vi "Main_C8855-01.vi"() -> ()   [LabVIEW 2017]
uses:
  C8855_MainD.ctl
  C8855-01api.dll
panel:
  in  "TrgEdge":u8(ring) caption="Trigger Edge"
  in  "TrgMode":u8(ring) caption="Trigger Mode" items=["SOFTWARE", "EXTERNAL"]
  out "Continue":bool
  in  "SStop":bool caption="Start"
  out "Gstep":dbl
  out "RR2":u8
  out "RR1":u8
  out "Moni2":string caption="Monitor CH2 [s^-1]"
  in  "Monitor":bool caption="Start"
  in  "Exit":bool caption="Start"
  in  "Load":bool caption="Start"
  in  "Save":bool caption="Start"
  in  "Start":bool
  in  "Tab":enum32{"CH1", "CH2"}(tab)
  in  "Power":bool caption="ブール"
  in  "OP10":bool caption="Outport 0"
  in  "OP11":bool caption="Outport 1"
  out "ID1":u8 caption="ID Code"
  in  "OP21":bool caption="Outport 1"
  in  "OP20":bool caption="Outport 0"
  in  "Power2":bool caption="ブール"
  out "ID2":u8 caption="ID Code"
  in  "MainD":T1 {"G_DIM" format="%.5f"}
  in  "Real":bool=TRUE caption="Real Time Display"
  out "Moni1":string caption="Monitor CH1 [s^-1]"
  out "Error":bool
  in  "LIN_Log":bool
  out "MT":dbl caption="Measurement \nTimes[sec]" format="%#.5f"
  in  "MP":u32=100 caption="Measurment \nPoints" min=10 max=100000
  in  "GT":i32(ring)=4 caption="Gate Time" items=["50 us", "100 us", "200 us", "500 us", "1 ms", "2 ms", "5 ms", "10 ms", "20 ms", "50 ms", "100 ms", "200 ms", "500ms", "1 s", "2 s", "5 s", "10 s"]
  out "Graph":cluster{dbl, dbl, u32[][]}(graph)
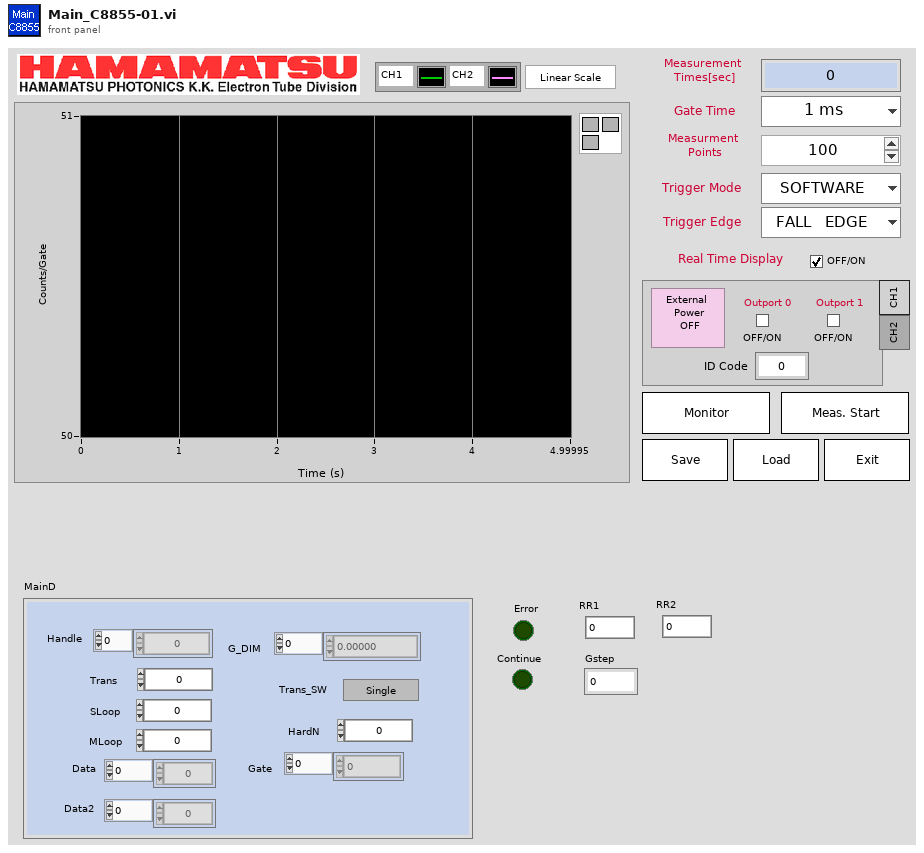
[diagram p1: front panel]
types:
  T1 = typedef "C8855_MainD.ctl" = cluster{"Handle":i64[], "G_DIM":dbl[], "Trans":u16, "Trans_SW":bool, "HardN":i32, "Gate":u8[], "Data":u32[], "Data2":u32[], "SLoop":i32, "MLoop":i32}
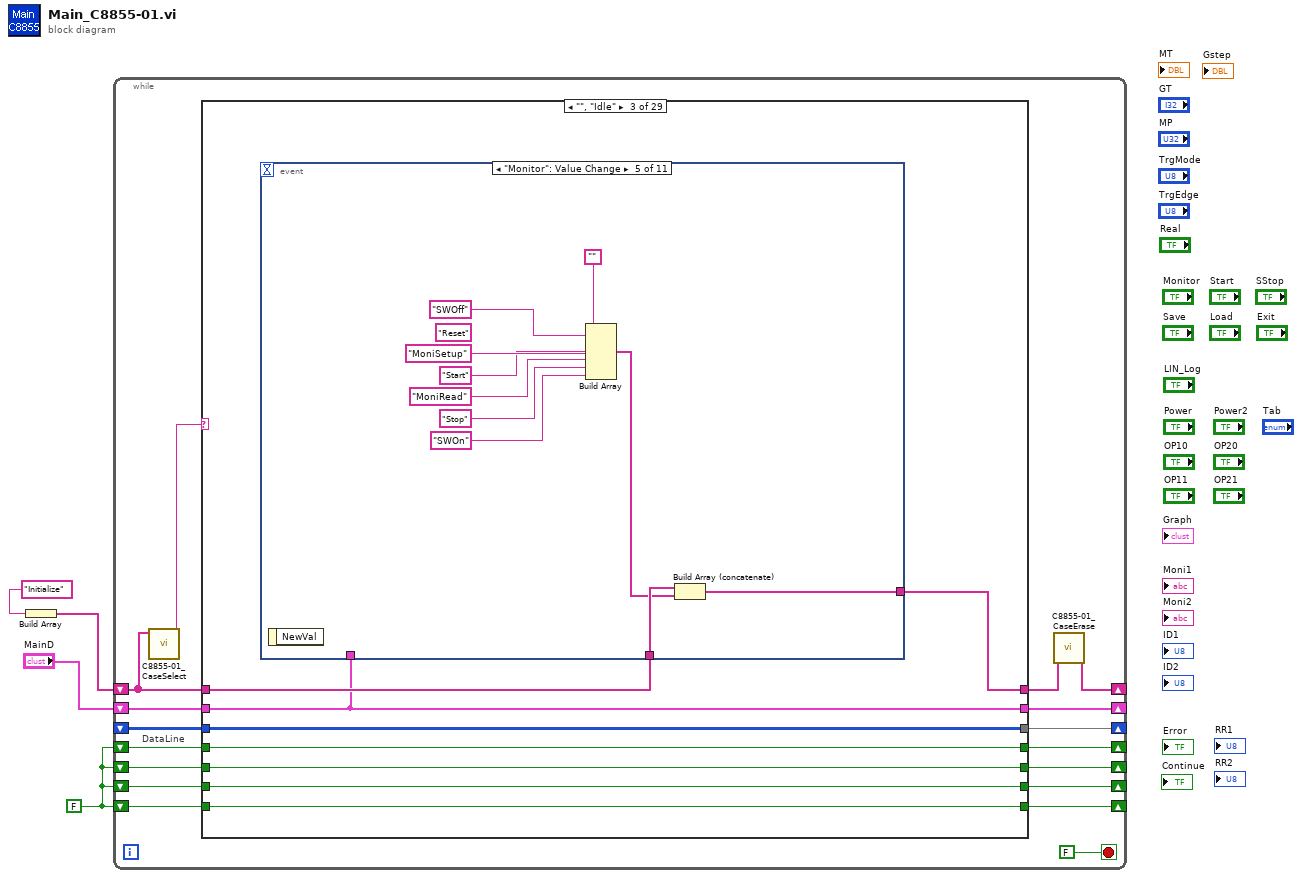
[diagram p0: block diagram]
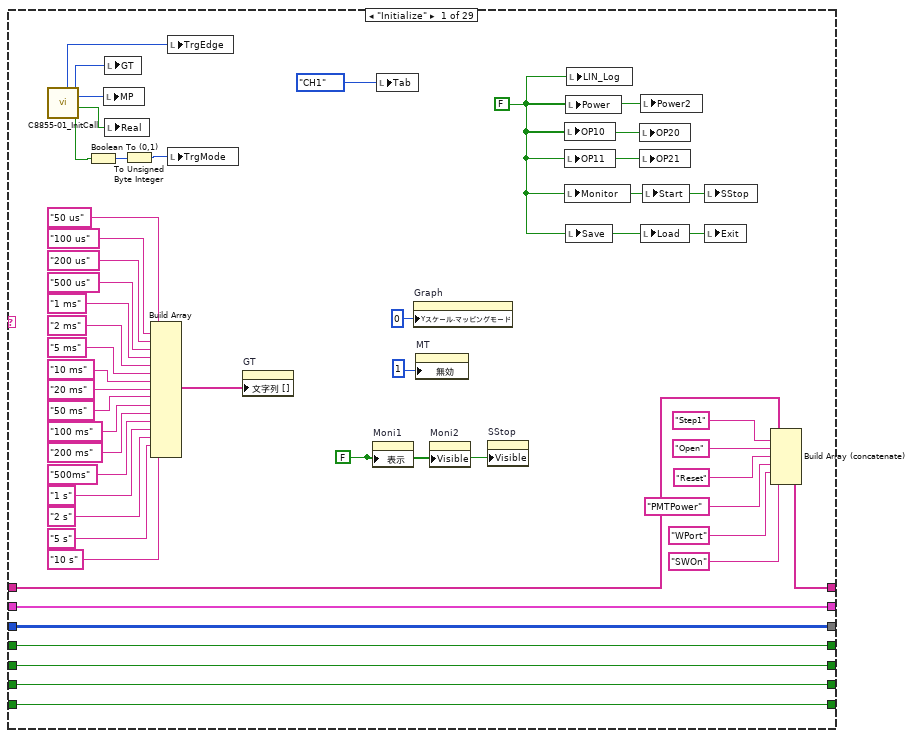
[diagram p2: hidden frame]
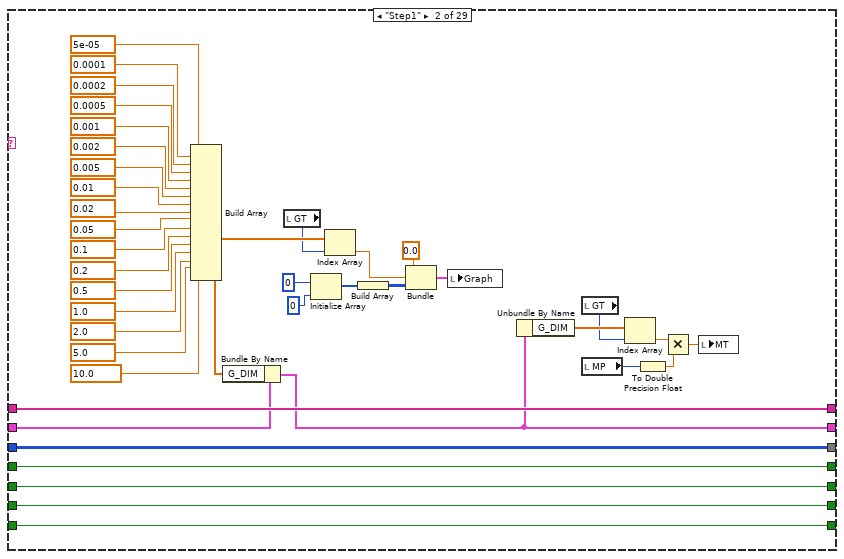
[diagram p3: hidden frame]
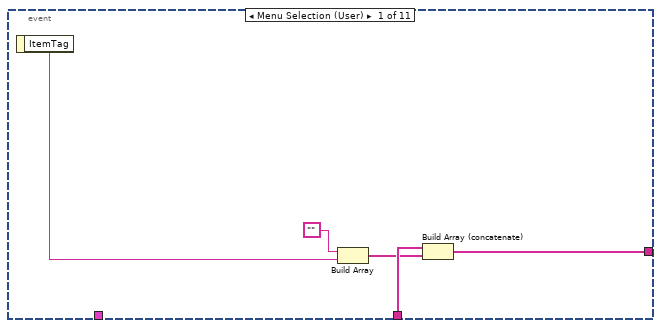
[diagram p4: hidden frame]
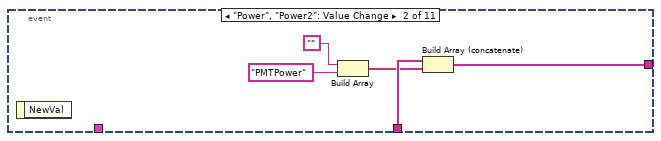
[diagram p5: hidden frame]
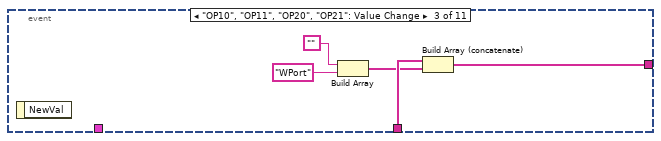
[diagram p6: hidden frame]
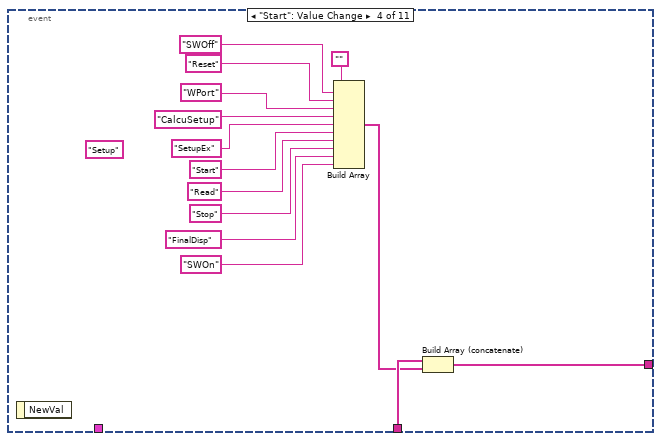
[diagram p7: hidden frame]
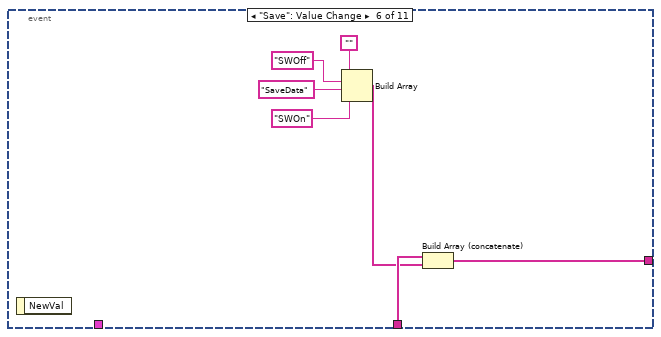
[diagram p8: hidden frame]
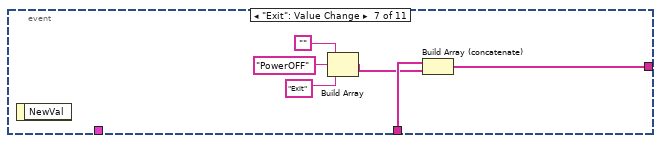
[diagram p9: hidden frame]
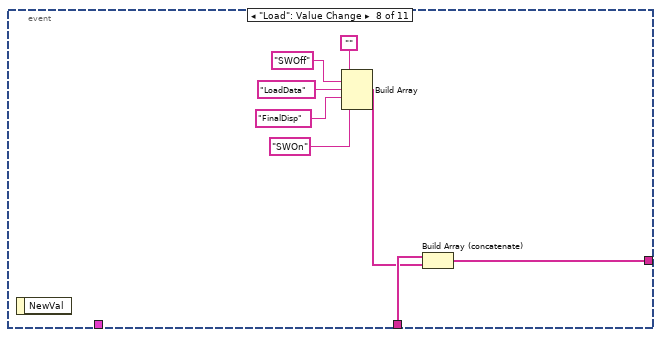
[diagram p10: hidden frame]
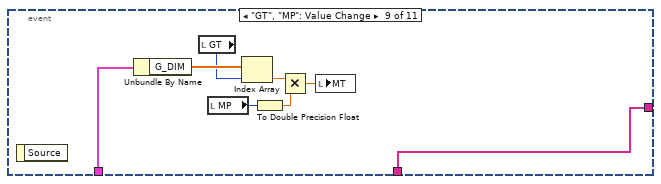
[diagram p11: hidden frame]
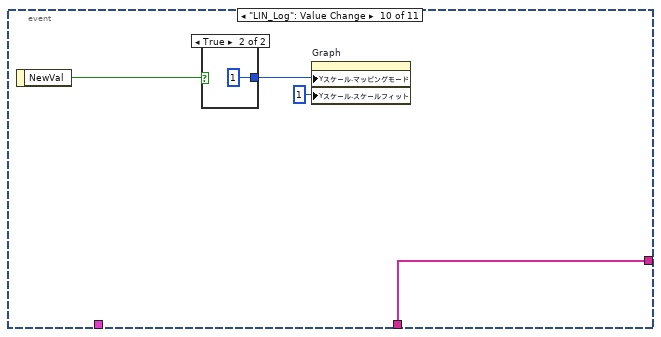
[diagram p12: hidden frame]
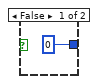
[diagram p13: hidden frame]
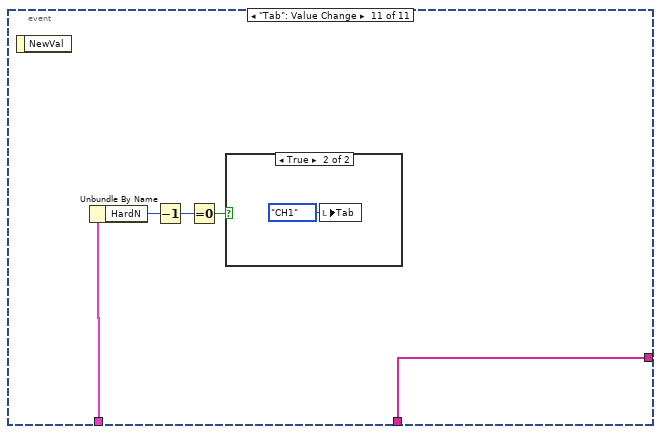
[diagram p14: hidden frame]
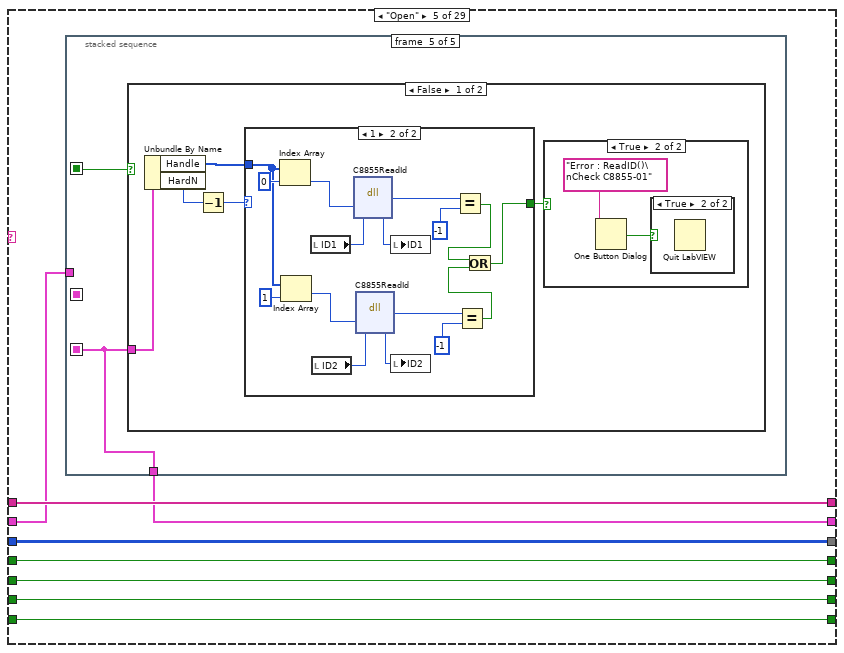
[diagram p17: hidden frame]
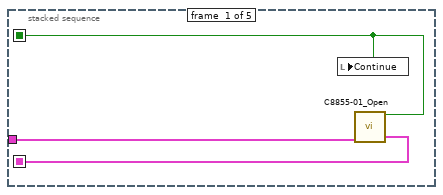
[diagram p18: hidden frame]
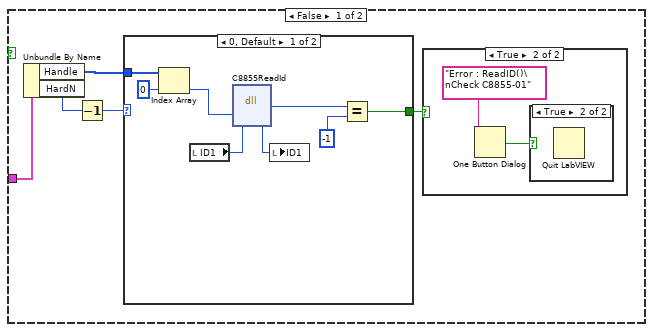
[diagram p20: hidden frame]
diagram:
  w3 = FALSE
  n1 = Build Array("Initialize") -> (w1:string[])
  n2 = while {
    shift-right: [w16] -> _
    shift-left: w3 -> [w17]
    shift-right: [w14] -> _
    shift-left: w3 -> [w15]
    shift-right: [w12] -> _
    shift-left: _ -> [w13]
    shift-right: [w10] -> _
    shift-left: "MainD" -> [w11]
    shift-right: [w5] -> _
    shift-left: w1 -> [w9]
    shift-right: [w18] -> _
    shift-left: w3 -> [w19]
    shift-right: [w20] -> _
    shift-left: w3 -> [w21]
    stop <- FALSE stop-if-true
    # "DataLine"
    n3 = call "C8855-01_CaseSelect.vi"("Input"=w9) -> ("Case"=w7:string)  [unwired: 10 out]
    n4 = case shown="\"\", \"Idle\"" w7 {
      tunnel: w21 -> [w65 w105 w113 w200 w208 w313 w335 w342 w369 w408 w440 w635 w670 w681 w698 w717 w774 w785 w800 w817 w831 w844 w883 w931 w963 w970 w977 w991 w998]
      tunnel: [w65 w105 w113 w200 w208 w313 w335 w342 w369 w408 w440 w635 w670 w681 w698 w717 w774 w785 w800 w817 w831 w844 w883 w931 w963 w970 w977 w991 w998] -> w20
      tunnel: w19 -> [w64 w104 w112 w199 w207 w312 w334 w341 w368 w407 w439 w634 w669 w680 w697 w716 w773 w784 w799 w816 w830 w843 w882 w930 w962 w969 w976 w990 w997]
      tunnel: [w64 w104 w112 w199 w207 w312 w334 w341 w368 w407 w439 w634 w669 w680 w697 w716 w773 w784 w799 w816 w830 w843 w882 w930 w962 w969 w976 w990 w997] -> w18
      tunnel: w17 -> [w63 w103 w111 w198 w206 w311 w333 w340 w367 w406 w438 w633 w668 w679 w696 w715 w772 w783 w798 w815 w829 w842 w881 w929 w961 w968 w975 w989 w996]
      tunnel: [w63 w103 w111 w198 w206 w311 w333 w340 w367 w406 w438 w633 w668 w679 w696 w715 w772 w783 w798 w815 w829 w842 w881 w929 w961 w968 w975 w989 w996] -> w16
      tunnel: w15 -> [w62 w102 w110 w197 w205 w310 w332 w339 w366 w405 w437 w632 w667 w678 w695 w714 w771 w782 w797 w814 w828 w841 w880 w928 w960 w967 w974 w988 w995]
      tunnel: [w62 w102 w110 w197 w205 w310 w332 w339 w366 w405 w437 w632 w667 w678 w695 w714 w771 w782 w797 w814 w828 w841 w880 w928 w960 w967 w974 w988 w995] -> w14
      tunnel: w13 -> [w61 w101 w109 w196 w204 w309 w331 w338 w365 w404 _ w631 w653 w677 w694 w713 w770 w781 w796 w813 w827 w840 w879 w920 w959 w966 w973 w987 w994]
      tunnel: [w61 w101 w109 w196 w204 w309 w331 w338 w365 w404 w428 w631 w653 w677 w694 w713 w770 w781 w796 w813 w827 w840 w879 w921 w959 w966 w973 w987 w994] -> w12
      tunnel: w11 -> [w29 w82 w106 w195 w202 w307 w322 w336 w363 w402 w434 w630 w665 w676 w687 w711 w769 w780 w795 w811 w825 w838 w878 w913 w958 w964 w971 w986 w992]
      tunnel: [w29 w67 w106 w195 w201 w307 w329 w336 w363 w402 w432 w630 w665 w676 w686 w711 w769 w780 w795 w811 w825 w838 w878 w913 w958 w964 w971 w986 w992] -> w10
      tunnel: w9 -> [w36 w100 w108 w194 w203 w308 w330 w337 w364 w403 w430 w624 w666 w675 w693 w712 w768 w779 w794 w812 w826 w839 w877 w927 w957 w965 w972 w984 w993]
      tunnel: [w35 w100 w107 w194 w203 w308 w330 w337 w364 w403 w429 w624 w666 w675 w693 w712 w768 w779 w794 w812 w826 w839 w877 w927 w957 w965 w972 w984 w993] -> w6
      frame "Initialize" {
        w27 = FALSE ("表示")
        w26 = FALSE ("Power")
        n5 = call "C8855-01_InitCall.vi"() -> ("ExtT"=w25:bool, "Moni"=w40:bool, "Measur"=w31:u32, "GT"=w30:i32, "TrgEdge"=w22:u8)  [unwired: 6 out]
        n6 = Boolean To (0,1)(Boolean=w25) -> (0, 1=w24:i16)
        n7 = local write "MP"(w31) -> ()
        n8 = local write "GT"(w30) -> ()
        n9 = local write "Real"(w40) -> ()
        n10 = To Unsigned Byte Integer(number=w24) -> (unsigned 8bit integer=w23:u8)
        n11 = Build Array("50 us", "100 us", "200 us", "500 us", "1 ms", "2 ms", "5 ms", "10 ms", "20 ms", "50 ms", "100 ms", "200 ms", "500ms", "1 s", "2 s", "5 s", "10 s") -> (w59:string[])
        n12 = local write "TrgEdge"(w22) -> ()
        n13 = local write "TrgMode"(w23) -> ()
        n14 = property on="GT" class="Ring (strict)"("文字列 []"=w59) -> ()  [unwired: 2 in, 2 out]
        n15 = property on="Moni1" class="Str"("表示"=w27) -> ()  [unwired: 2 in, 2 out]
        n16 = local write "Tab"(enum32{"CH1", "CH2"}."CH1" ("Tab")) -> ()
        n17 = property on="Graph" class="WFGraph (strict)"("Yスケール.マッピングモード"=u8 0 ("Y Scale.Mapping Mode")) -> ()  [unwired: 2 in, 2 out]
        n18 = property on="MT" class="DigNum (strict)"("無効"=u8 1 ("Disabled")) -> ()  [unwired: 2 in, 2 out]
        n19 = property on="Moni2" class="Str"("Visible"=w27) -> ()  [unwired: 2 in, 2 out]
        n20 = property on="SStop" class="Bool (strict)"("Visible"=w27) -> ()  [unwired: 2 in, 2 out]
        n21 = local write "OP10"(w26) -> ()
        n22 = local write "OP11"(w26) -> ()
        n23 = local write "Monitor"(w26) -> ()
        n24 = local write "Power"(w26) -> ()
        n25 = local write "Save"(w26) -> ()
        n26 = local write "LIN_Log"(w26) -> ()
        n27 = local write "OP20"(w26) -> ()
        n28 = local write "OP21"(w26) -> ()
        n29 = local write "Power2"(w26) -> ()
        n30 = local write "Load"(w26) -> ()
        n31 = local write "Start"(w26) -> ()
        n32 = local write "SStop"(w26) -> ()
        n33 = local write "Exit"(w26) -> ()
        n34 = Build Array (concatenate)(w36, "Step1", "Open", "Reset", "PMTPower", "WPort", "SWOn") -> (w35:string[])
      }
      frame "Step1" {
        n35 = Build Array(5e-05, 0.0001, 0.0002, 0.0005, 0.001, 0.002, 0.005, 0.01, 0.02, 0.05, 0.1, 0.2, 0.5, 1.0, 2.0, 5.0, 10.0) -> (w77:dbl[])
        n36 = Bundle By Name(cluster=w82, "G_DIM"=w77) -> (w67:T1)
        n37 = local read "GT"() -> (w76:i32)
        n38 = Initialize Array(u32 0 ("element"), 0 ("dimension size")) -> (w81:u32[])
        n39 = Index Array(array=w77, index=w76) -> (element=w75:dbl)
        n40 = Build Array(w81) -> (w74:u32[][])
        n41 = Bundle(0.0, w75, w74) -> (w66:cluster{dbl, dbl, u32[][]})  [unwired: 1 out]
        n42 = local write "Graph"(w66) -> ()
        n43 = Unbundle By Name(w67) -> ("G_DIM"=w70:dbl[])
        n44 = local read "GT"() -> (w69:i32)
        n45 = local read "MP"() -> (w72:u32)
        n46 = Index Array(array=w70, index=w69) -> (element=w73:dbl)
        n47 = To Double Precision Float(number=w72) -> (double precision float=w71:dbl)
        n48 = Multiply(x=w73, y=w71) -> (x*y=w68:dbl)
        n49 = local write "MT"(w68) -> ()
      }
      frame "", "Idle" {
        n50 = event shown="[4] \"Monitor\": Value Change" {
          selector: _ -> [_ _ _ _ _ _ _ _ _ _ _]
          dyn-events: _ -> [_ _ _ _ _ _ _ _ _ _ _]
          timeout: _ -> [_ _ _ _ _ _ _ _ _ _ _]
          tunnel: w108 -> [w116 w122 w127 w142 w152 w159 w165 w173 w174 w182 w192]
          tunnel: [w114 w120 w125 w140 w150 w157 w163 w171 w174 w182 w192] -> w107
          tunnel: w106 -> [_ _ _ _ _ _ _ _ w175 _ w191]
          event Menu Selection (User) {
            n51 = event-data() -> ("ItemTag"=w117:string)  [unwired: 1 out]
            n52 = Build Array("", w117) -> (w115:string[])
            n53 = Build Array (concatenate)(w116, w115) -> (w114:string[])
          }
          event "Power", "Power2": Value Change {
            n54 = event-data() -> ()  [unwired: 2 out]
            n55 = Build Array("", "PMTPower" ("要素")) -> (w121:string[])
            n56 = Build Array (concatenate)(w122, w121) -> (w120:string[])
          }
          event "OP10", "OP11", "OP20", "OP21": Value Change {
            n57 = event-data() -> ()  [unwired: 2 out]
            n58 = Build Array("", "WPort" ("要素")) -> (w126:string[])
            n59 = Build Array (concatenate)(w127, w126) -> (w125:string[])
          }
          event "Start": Value Change {
            (unwired) "Setup" ("要素")
            n60 = event-data() -> ()  [unwired: 2 out]
            n61 = Build Array("", "SWOff" ("要素"), "Reset" ("要素"), "WPort" ("要素"), "CalcuSetup" ("要素"), "SetupEx" ("要素"), "Start" ("要素"), "Read" ("要素"), "Stop" ("要素"), "FinalDisp" ("要素"), "SWOn" ("要素")) -> (w141:string[])
            n62 = Build Array (concatenate)(w142, w141) -> (w140:string[])
          }
          event "Monitor": Value Change {
            (unwired) "Reset" ("要素")
            n63 = event-data() -> ()  [unwired: 2 out]
            n64 = Build Array("", "SWOff" ("要素"), "MoniSetup" ("要素"), "Start" ("要素"), "MoniRead" ("要素"), "Stop" ("要素"), "SWOn" ("要素")) -> (w151:string[])
            n65 = Build Array (concatenate)(w152, w151) -> (w150:string[])
          }
          event "Save": Value Change {
            n66 = event-data() -> ()  [unwired: 2 out]
            n67 = Build Array("", "SWOff" ("要素"), "SaveData" ("要素"), "SWOn" ("要素")) -> (w158:string[])
            n68 = Build Array (concatenate)(w159, w158) -> (w157:string[])
          }
          event "Exit": Value Change {
            n69 = event-data() -> ()  [unwired: 2 out]
            n70 = Build Array("", "PowerOFF" ("要素"), "Exit" ("要素")) -> (w164:string[])
            n71 = Build Array (concatenate)(w165, w164) -> (w163:string[])
          }
          event "Load": Value Change {
            n72 = event-data() -> ()  [unwired: 2 out]
            n73 = Build Array("", "SWOff" ("要素"), "LoadData" ("要素"), "FinalDisp" ("要素"), "SWOn" ("要素")) -> (w172:string[])
            n74 = Build Array (concatenate)(w173, w172) -> (w171:string[])
          }
          event "GT", "MP": Value Change {
            n75 = event-data() -> ()  [unwired: 2 out]
            n76 = Unbundle By Name(w175) -> ("G_DIM"=w178:dbl[])
            n77 = local read "GT"() -> (w177:i32)
            n78 = local read "MP"() -> (w180:u32)
            n79 = Index Array(array=w178, index=w177) -> (element=w181:dbl)
            n80 = To Double Precision Float(number=w180) -> (double precision float=w179:dbl)
            n81 = Multiply(x=w181, y=w179) -> (x*y=w176:dbl)
            n82 = local write "MT"(w176) -> ()
          }
          event "LIN_Log": Value Change {
            n83 = event-data() -> ("NewVal"=w183:bool)  [unwired: 1 out]
            n84 = case shown="True" w183 {
              tunnel: [u8 0 ("Yスケール.マッピングモード") u8 1 ("Yスケール.マッピングモード")] -> w184
              frame False {
              }
              frame True {
              }
            }
            n85 = property on="Graph" class="WFGraph (strict)"("Yスケール.マッピングモード"=w184, "Yスケール.スケールフィット"=u8 1 ("Y Scale.Scale Fit")) -> ()  [unwired: 2 in, 2 out]
          }
          event "Tab": Value Change {
            n86 = event-data() -> ()  [unwired: 2 out]
            n87 = Unbundle By Name(w191) -> ("HardN"=w190:i32)
            n88 = Decrement(x=w190) -> (x-1=w189:i32)
            n89 = Equal To 0?(x=w189) -> (x = 0?=w188:bool)
            n90 = case shown="True" w188 {
              frame False {
              }
              frame True {
                n91 = local write "Tab"(enum32{"CH1", "CH2"}."CH1" ("Tab")) -> ()
              }
            }
          }
        }
      }
      frame "//////////////" {
      }
      frame "Open" {
        n92 = stacked-sequence {
          seq-local: [w210 _ _ _ _] -> [_ w213 w246 w259 _]
          seq-local: [_ _ _ w258 _] -> [_ _ _ _ w280]
          seq-local: [w209 _ _ _ _] -> [_ w212 w245 w257 w281]
          tunnel: w202 -> [w211 _ _ _ _]
          tunnel: [_ _ _ _ w280] -> w201
          frame #0 {
            n93 = call "C8855-01_Open.vi"("MainD"=w211) -> ("Continue"=w209:bool, "MainDR"=w210:T1)  [unwired: 1 in, 12 out]
            n94 = local write "Continue"(w209) -> ()
          }
          frame #1 {
            n95 = case shown="True" w212 {
              tunnel: w213 -> [w214 _]
              frame False {
                n96 = Unbundle By Name(w214) -> ("Handle"=w216:i64[], "HardN"=w218:i32)
                n97 = Decrement(x=w218) -> (x-1=w217:i32)
                n98 = case shown="0, Default" w217 {
                  tunnel: w216 -> [w228 w237]
                  tunnel: [w222 w229] -> w215
                  frame 0, Default {
                    n99 = Index Array(array=w228, index=0 ("指標")) -> (element=w226:i64)
                    n100 = local read "ID1"() -> (w225:u8)
                    n101 = dll-call lib="PTH2³unc \\\\den0\\é›»å¿œã‚·ã‚¹ãƒ†ãƒ éƒ¨é›»å¿œã‚·ã‚¹ãƒ†ãƒ éƒ¨å†…è³‡æ–™13éƒ¨é–€33412â–  C8855-01â–¡ä»˜å±žï¼£ï¼¤C8855-01 Ver3.4[æœ€æ–°]SampleSourcex64C8855-01api.dll" fn="C8855ReadId"("Handle"=w226, "ID"=w225) -> ("返り値タイプ"=w221:i32, "ID"=w224:u8)  [unwired: 4 in, 2 out]
                    n102 = local write "ID1"(w224) -> ()
                    n103 = Equal?(x=w221, y=-1) -> (x = y?=w222:bool)
                  }
                  frame 1 {
                    n104 = Index Array(array=w237, index=0 ("指標")) -> (element=w243:i64)
                    n105 = Index Array(array=w237, index=1 ("指標")) -> (element=w238:i64)
                    n106 = local read "ID1"() -> (w242:u8)
                    n107 = local read "ID2"() -> (w236:u8)
                    n108 = dll-call lib="PTH2³unc \\\\den0\\é›»å¿œã‚·ã‚¹ãƒ†ãƒ éƒ¨é›»å¿œã‚·ã‚¹ãƒ†ãƒ éƒ¨å†…è³‡æ–™13éƒ¨é–€33412â–  C8855-01â–¡ä»˜å±žï¼£ï¼¤C8855-01 Ver3.4[æœ€æ–°]SampleSourcex64C8855-01api.dll" fn="C8855ReadId"("Handle"=w243, "ID"=w242) -> ("返り値タイプ"=w234:i32, "ID"=w241:u8)  [unwired: 4 in, 2 out]
                    n109 = dll-call lib="PTH2³unc \\\\den0\\é›»å¿œã‚·ã‚¹ãƒ†ãƒ éƒ¨é›»å¿œã‚·ã‚¹ãƒ†ãƒ éƒ¨å†…è³‡æ–™13éƒ¨é–€33412â–  C8855-01â–¡ä»˜å±žï¼£ï¼¤C8855-01 Ver3.4[æœ€æ–°]SampleSourcex64C8855-01api.dll" fn="C8855ReadId"("Handle"=w238, "ID"=w236) -> ("返り値タイプ"=w233:i32, "ID"=w235:u8)  [unwired: 4 in, 2 out]
                    n110 = local write "ID1"(w241) -> ()
                    n111 = local write "ID2"(w235) -> ()
                    n112 = Equal?(x=w234, y=-1) -> (x = y?=w230:bool)
                    n113 = Equal?(x=w233, y=-1) -> (x = y?=w231:bool)
                    n114 = Or(x=w230, y=w231) -> (x .or. y?=w229:bool)
                  }
                }
                n115 = case shown="True" w215 {
                  frame False {
                  }
                  frame True {
                    n116 = One Button Dialog(message="Error : ReadID()\nCheck C8855-01" ("爷景嫁")) -> (true=w220:bool)  [unwired: 1 out]
                    n117 = case shown="True" w220 {
                      frame False {
                      }
                      frame True {
                        n118 = Quit LabVIEW() -> ()  [unwired: 1 out]
                      }
                    }
                  }
                }
              }
              frame True {
              }
            }
          }
          frame #2 {
            n119 = case shown="False" w245 {
              tunnel: w246 -> [w247 _]
              frame False {
                n120 = Unbundle By Name(w247) -> ("HardN"=w250:i32)
                n121 = Decrement(x=w250) -> (x-1=w249:i32)
                n122 = case shown="1" w249 {
                  tunnel: [FALSE w254] -> w248
                  frame 0, Default {
                  }
                  frame 1 {
                    n123 = local read "ID1"() -> (w256:u8)
                    n124 = local read "ID2"() -> (w255:u8)
                    n125 = Equal?(x=w256, y=w255) -> (x = y?=w254:bool)
                  }
                }
                n126 = case shown="True" w248 {
                  frame False {
                  }
                  frame True {
                    n127 = One Button Dialog(message="Error :ID overlaps. \nCheck C8855-01" ("爷景嫁")) -> (true=w252:bool)  [unwired: 1 out]
                    n128 = case shown="True" w252 {
                      frame False {
                      }
                      frame True {
                        n129 = Quit LabVIEW() -> ()  [unwired: 1 out]
                      }
                    }
                  }
                }
              }
              frame True {
              }
            }
          }
          frame #3 {
            n130 = case shown="False" w257 {
              tunnel: w259 -> [w261 w279]
              tunnel: [w260 w279] -> w258
              frame False {
                n131 = Unbundle By Name(w261) -> ("HardN"=w263:i32)
                n132 = Decrement(x=w263) -> (x-1=w262:i32)
                n133 = case shown="1" w262 {
                  tunnel: w261 -> [w264 w266]
                  tunnel: [w264 w265] -> w260
                  frame 0, Default {
                  }
                  frame 1 {
                    n134 = local read "ID1"() -> (w269:u8)
                    n135 = local read "ID2"() -> (w268:u8)
                    n136 = Greater?(x=w269, y=w268) -> (0:w267:bool)
                    n137 = case shown="False" w267 {
                      tunnel: w266 -> [w270 w275]
                      tunnel: [w270 w271] -> w265
                      frame False {
                      }
                      frame True {
                        n138 = Unbundle By Name(w275) -> ("Handle"=w278:i64[])
                        n139 = Index Array(array=w278, index=0 ("指標")) -> (element=w274:i64)
                        n140 = Index Array(array=w278, index=1 ("指標")) -> (element=w273:i64)
                        n141 = Build Array(w273, w274) -> (w272:i64[])
                        n142 = Bundle By Name(cluster=w275, "Handle"=w272) -> (w271:T1)
                      }
                    }
                  }
                }
              }
              frame True {
              }
            }
          }
          frame #4 {
            n143 = case shown="False" w281 {
              tunnel: w280 -> [w282 _]
              frame False {
                n144 = Unbundle By Name(w282) -> ("Handle"=w284:i64[], "HardN"=w286:i32)
                n145 = Decrement(x=w286) -> (x-1=w285:i32)
                n146 = case shown="1" w285 {
                  tunnel: w284 -> [_ w298]
                  tunnel: [FALSE w290] -> w283
                  frame 0, Default {
                  }
                  frame 1 {
                    n147 = Index Array(array=w298, index=0 ("指標")) -> (element=w304:i64)
                    n148 = Index Array(array=w298, index=1 ("指標")) -> (element=w299:i64)
                    n149 = local read "ID1"() -> (w303:u8)
                    n150 = local read "ID2"() -> (w297:u8)
                    n151 = dll-call lib="PTH2³unc \\\\den0\\é›»å¿œã‚·ã‚¹ãƒ†ãƒ éƒ¨é›»å¿œã‚·ã‚¹ãƒ†ãƒ éƒ¨å†…è³‡æ–™13éƒ¨é–€33412â–  C8855-01â–¡ä»˜å±žï¼£ï¼¤C8855-01 Ver3.4[æœ€æ–°]SampleSourcex64C8855-01api.dll" fn="C8855ReadId"("Handle"=w304, "ID"=w303) -> ("返り値タイプ"=w295:i32, "ID"=w302:u8)  [unwired: 4 in, 2 out]
                    n152 = dll-call lib="PTH2³unc \\\\den0\\é›»å¿œã‚·ã‚¹ãƒ†ãƒ éƒ¨é›»å¿œã‚·ã‚¹ãƒ†ãƒ éƒ¨å†…è³‡æ–™13éƒ¨é–€33412â–  C8855-01â–¡ä»˜å±žï¼£ï¼¤C8855-01 Ver3.4[æœ€æ–°]SampleSourcex64C8855-01api.dll" fn="C8855ReadId"("Handle"=w299, "ID"=w297) -> ("返り値タイプ"=w294:i32, "ID"=w296:u8)  [unwired: 4 in, 2 out]
                    n153 = local write "ID1"(w302) -> ()
                    n154 = local write "ID2"(w296) -> ()
                    n155 = Equal?(x=w295, y=-1) -> (x = y?=w291:bool)
                    n156 = Equal?(x=w294, y=-1) -> (x = y?=w292:bool)
                    n157 = Or(x=w291, y=w292) -> (x .or. y?=w290:bool)
                  }
                }
                n158 = case shown="True" w283 {
                  frame False {
                  }
                  frame True {
                    n159 = One Button Dialog(message="Error : ReadID()\nCheck C8855-01" ("爷景嫁")) -> (true=w288:bool)  [unwired: 1 out]
                    n160 = case shown="True" w288 {
                      frame False {
                      }
                      frame True {
                        n161 = Quit LabVIEW() -> ()  [unwired: 1 out]
                      }
                    }
                  }
                }
              }
              frame True {
              }
            }
          }
        }
      }
      frame "Reset" {
        n162 = Unbundle By Name(w307) -> ("Handle"=w306:i64[])
        n163 = for {
          tunnel: w306 -> [w316] mode=indexing
          n164 = dll-call lib="PTH2³unc \\\\den0\\é›»å¿œã‚·ã‚¹ãƒ†ãƒ éƒ¨é›»å¿œã‚·ã‚¹ãƒ†ãƒ éƒ¨å†…è³‡æ–™13éƒ¨é–€33412â–  C8855-01â–¡ä»˜å±žï¼£ï¼¤C8855-01 Ver3.4[æœ€æ–°]SampleSourcex64C8855-01api.dll" fn="C8855Reset"("Hnadle"=w316) -> ("返り値タイプ"=w315:i32)  [unwired: 4 in, 2 out]
          n165 = Less Or Equal To 0?(x=w315) -> (x <= 0?=w314:bool)
          n166 = case shown="True" w314 {
            frame False {
            }
            frame True {
              n167 = One Button Dialog(message="Error : Reset()\nCheck C8855-01" ("爷景嫁")) -> (true=w317:bool)  [unwired: 1 out]
              n168 = case shown="True" w317 {
                frame False {
                }
                frame True {
                  n169 = Quit LabVIEW() -> ()  [unwired: 1 out]
                }
              }
            }
          }
        }
      }
      frame "CalcuSetup" {
        n170 = Unbundle By Name(w322) -> ("G_DIM"=w321:dbl[])
        n171 = local read "MP"() -> (w325:u32)
        n172 = local read "GT"() -> (w320:i32)
        n173 = call "C8855-01_CalcuP.vi"("MainD"=w322, "MP"=w325, "GT"=w320) -> ("MainDR"=w324:T1)  [unwired: 8 out]
        n174 = Index Array(array=w321, index=w320) -> (element=w319:dbl)
        n175 = local write "Gstep"(w319) -> ()
        n176 = Unbundle By Name(w324) -> ("Trans"=w323:u16)
        n177 = To Long Integer(number=w323) -> (32bit integer=w327:i32)
        n178 = Initialize Array(u32 0 ("element"), w327) -> (w326:u32[])
        n179 = Bundle By Name(cluster=w324, "Data"=w326, "Data2"=w326) -> (w329:T1)
      }
      frame "Setup" {
        n180 = stacked-sequence {
          tunnel: w336 -> [w348 _]
          frame #0 {
            n181 = Unbundle By Name(w348) -> ("Handle"=w347:i64[], "Gate"=w346:u8[], "Trans"=w344:u16)
            n182 = local read "GT"() -> (w345:i32)
            n183 = Index Array(array=w346, index=w345) -> (element=w343:u8)
            n184 = for {
              tunnel: w347 -> [w353] mode=indexing
              tunnel: w344 -> [w351]
              tunnel: w343 -> [w352]
              n185 = dll-call lib="PTH2³unc \\\\den0\\é›»å¿œã‚·ã‚¹ãƒ†ãƒ éƒ¨é›»å¿œã‚·ã‚¹ãƒ†ãƒ éƒ¨å†…è³‡æ–™13éƒ¨é–€33412â–  C8855-01â–¡ä»˜å±žï¼£ï¼¤C8855-01 Ver3.4[æœ€æ–°]SampleSourcex64C8855-01api.dll" fn="C8855Setup"("Handle"=w353, "Gatetime"=w352, "Transmode"=u8 2, "Number of gate"=w351) -> ("返り値タイプ"=w350:i32)  [unwired: 7 in, 2 out]
              n186 = Less Or Equal To 0?(x=w350) -> (x <= 0?=w349:bool)
              n187 = case shown="True" w349 {
                frame False {
                }
                frame True {
                  n188 = One Button Dialog(message="Error : Setup()\nCheck C8855-01" ("爷景嫁")) -> (true=w355:bool)  [unwired: 1 out]
                  n189 = case shown="True" w355 {
                    frame False {
                    }
                    frame True {
                      n190 = Quit LabVIEW() -> ()  [unwired: 1 out]
                    }
                  }
                }
              }
            }
          }
          frame #1 {
            n191 = local read "TrgEdge"() -> (w357:u8)
            n192 = local read "TrgMode"() -> (w361:u8)
            n193 = local read "MP"() -> (w359:u32)
            n194 = local read "GT"() -> (w358:i32)
            n195 = local read "Real"() -> (w360:bool)
            n196 = Greater Than 0?(x=w361) -> (x > 0?=w362:bool)
            n197 = call "C8855-01_InitWrite.vi"("TrgEdge"=w357, "ExtT"=w362, "Moni"=w360, "MP"=w359, "GT"=w358) -> ()  [unwired: 6 out]
          }
        }
      }
      frame "SetupEx" {
        n198 = stacked-sequence {
          tunnel: w363 -> [w376 _]
          frame #0 {
            n199 = Unbundle By Name(w376) -> ("Handle"=w375:i64[], "Gate"=w374:u8[], "Trans"=w372:u16)
            n200 = local read "TrgEdge"() -> (w370:u8)
            n201 = local read "GT"() -> (w373:i32)
            n202 = Index Array(array=w374, index=w373) -> (element=w371:u8)
            n203 = for {
              tunnel: w375 -> [w382] mode=indexing
              tunnel: w372 -> [w380]
              tunnel: w371 -> [w381]
              tunnel: w370 -> [w377]
              n204 = dll-call lib="PTH2³unc \\\\den0\\é›»å¿œã‚·ã‚¹ãƒ†ãƒ éƒ¨é›»å¿œã‚·ã‚¹ãƒ†ãƒ éƒ¨å†…è³‡æ–™13éƒ¨é–€33412â–  C8855-01â–¡ä»˜å±žï¼£ï¼¤C8855-01 Ver3.4[æœ€æ–°]SampleSourcex64C8855-01api.dll" fn="C8855SetupEx"("Handle"=w382, "Gatetime"=w381, "Transmode"=u8 2, "Number of gate"=w380, "TriggerEdge"=w377) -> ("返り値タイプ"=w379:i32)  [unwired: 8 in, 2 out]
              n205 = Less Or Equal To 0?(x=w379) -> (x <= 0?=w378:bool)
              n206 = case shown="True" w378 {
                frame False {
                }
                frame True {
                  n207 = One Button Dialog(message="Error : Setup()\nCheck C8855-01" ("爷景嫁")) -> (true=w384:bool)  [unwired: 1 out]
                  n208 = case shown="True" w384 {
                    frame False {
                    }
                    frame True {
                      n209 = Quit LabVIEW() -> ()  [unwired: 1 out]
                    }
                  }
                }
              }
            }
          }
          frame #1 {
            n210 = local read "TrgMode"() -> (w390:u8)
            n211 = local read "TrgEdge"() -> (w386:u8)
            n212 = local read "MP"() -> (w388:u32)
            n213 = local read "GT"() -> (w387:i32)
            n214 = local read "Real"() -> (w389:bool)
            n215 = Greater Than 0?(x=w390) -> (x > 0?=w391:bool)
            n216 = call "C8855-01_InitWrite.vi"("TrgEdge"=w386, "ExtT"=w391, "Moni"=w389, "MP"=w388, "GT"=w387) -> ()  [unwired: 6 out]
          }
        }
      }
      frame "Start" {
        n217 = local read "Monitor"() -> (w392:bool)
        n218 = local read "TrgMode"() -> (w395:u8)
        n219 = Unbundle By Name(w402) -> ("Handle"=w398:i64[], "HardN"=w401:i32)
        n220 = Decrement(x=w401) -> (x-1=w400:i32)
        n221 = Select(t=u8 0 ("Mode"), s=w392, f=w395) -> (s? t:f=w393:u8)
        n222 = Not Equal To 0?(x=w400) -> (x != 0?=w399:bool)
        n223 = case shown="True" w399 {
          tunnel: w398 -> [w419 w426]
          tunnel: w393 -> [w416 w424]
          tunnel: [w415 w422] -> w396
          frame True {
            n224 = Index Array(array=w419, index=1 ("指標")) -> (element=w421:i64)
            n225 = Index Array(array=w419, index=0 ("指標")) -> (element=w420:i64)
            n226 = dll-call lib="PTH2³unc \\\\den0\\é›»å¿œã‚·ã‚¹ãƒ†ãƒ éƒ¨é›»å¿œã‚·ã‚¹ãƒ†ãƒ éƒ¨å†…è³‡æ–™13éƒ¨é–€33412â–  C8855-01â–¡ä»˜å±žï¼£ï¼¤C8855-01 Ver3.4[æœ€æ–°]SampleSourcex64C8855-01api.dll" fn="C8855CountStart"("Hnadle"=w421, "Mode"=w416) -> ("返り値タイプ"=w412:i32)  [unwired: 5 in, 2 out]
            n227 = dll-call lib="PTH2³unc \\\\den0\\é›»å¿œã‚·ã‚¹ãƒ†ãƒ éƒ¨é›»å¿œã‚·ã‚¹ãƒ†ãƒ éƒ¨å†…è³‡æ–™13éƒ¨é–€33412â–  C8855-01â–¡ä»˜å±žï¼£ï¼¤C8855-01 Ver3.4[æœ€æ–°]SampleSourcex64C8855-01api.dll" fn="C8855CountStart"("Hnadle"=w420, "Mode"=w416) -> ("返り値タイプ"=w414:i32)  [unwired: 5 in, 2 out]
            n228 = Less Or Equal To 0?(x=w414) -> (x <= 0?=w413:bool)
            n229 = Less Or Equal To 0?(x=w412) -> (x <= 0?=w411:bool)
            n230 = Or(x=w413, y=w411) -> (x .or. y?=w415:bool)
          }
          frame False {
            n231 = Index Array(array=w426, index=0 ("指標")) -> (element=w425:i64)
            n232 = dll-call lib="PTH2³unc \\\\den0\\é›»å¿œã‚·ã‚¹ãƒ†ãƒ éƒ¨é›»å¿œã‚·ã‚¹ãƒ†ãƒ éƒ¨å†…è³‡æ–™13éƒ¨é–€33412â–  C8855-01â–¡ä»˜å±žï¼£ï¼¤C8855-01 Ver3.4[æœ€æ–°]SampleSourcex64C8855-01api.dll" fn="C8855CountStart"("Hnadle"=w425, "Mode"=w424) -> ("返り値タイプ"=w423:i32)  [unwired: 5 in, 2 out]
            n233 = Less Or Equal To 0?(x=w423) -> (x <= 0?=w422:bool)
          }
        }
        n234 = local write "Error"(FALSE ("Error")) -> ()
        n235 = case shown="True" w396 {
          frame False {
          }
          frame True {
            n236 = One Button Dialog(message="Error : Start()\nCheck C8855-01" ("爷景嫁")) -> (true=w409:bool)  [unwired: 1 out]
            n237 = case shown="True" w409 {
              frame False {
              }
              frame True {
                n238 = Quit LabVIEW() -> ()  [unwired: 1 out]
              }
            }
          }
        }
      }
      frame "Read" {
        n239 = Unbundle By Name(w434) -> ("MLoop"=w431:i32, "SLoop"=w435:i32)
        n240 = Equal?(x=w435, y=1) -> (x = y?=w433:bool)
        n241 = case shown="False" w433 {
          tunnel: w435 -> [_ w550]
          tunnel: w434 -> [w447 w549]
          tunnel: [w446 w548] -> w432
          tunnel: w431 -> [w442 w546]
          tunnel: w430 -> [w444 w543]
          tunnel: [w443 w542] -> w429
          tunnel: [w441 w540] -> w428
          frame True {
            n242 = stacked-sequence {
              seq-local: [w449 _] -> [_ w525]
              seq-local: [w450 _] -> [_ w524]
              seq-local: [w448 _] -> [_ w529]
              tunnel: w447 -> [w455 _]
              tunnel: [_ w529] -> w446
              tunnel: [w452 _] -> w445
              tunnel: w442 -> [w451 _]
              tunnel: [_ w523] -> w441
              frame #0 {
                w454 = u32[] []
                n243 = for {
                  N: w451 -> [_]
                  shift-right: [w459] -> w449
                  shift-left: w454 -> [w461]
                  shift-right: [w458] -> w450
                  shift-left: w454 -> [w460]
                  shift-right: [w457] -> w448
                  shift-left: w455 -> [w463]
                  shift-right: [w462] -> w452
                  shift-left: FALSE -> [w456]
                  n244 = stacked-sequence {
                    seq-local: [w466 _ _] -> [_ w479 _]
                    seq-local: [w464 _ _] -> [_ w474 _]
                    seq-local: [_ w473 _] -> [_ _ w521]
                    tunnel: w463 -> [w467 _ _]
                    tunnel: w456 -> [w465 _ _]
                    tunnel: [_ _ w522] -> w462
                    tunnel: w461 -> [_ w478 _]
                    tunnel: w460 -> [_ w477 _]
                    tunnel: [_ w476 _] -> w459
                    tunnel: [_ w475 _] -> w458
                    tunnel: [_ w474 _] -> w457
                    frame #0 {
                      n245 = case shown="False" w465 {
                        selector: w465 -> [_ w472]
                        tunnel: w467 -> [w470 w471]
                        tunnel: [w469 w472] -> w466
                        tunnel: [w468 w471] -> w464
                        frame False {
                          n246 = call "C8855-01_ReadData.vi"("MainD"=w470) -> ("MainDR"=w468:T1, "Error"=w469:bool)  [unwired: 9 out]
                        }
                        frame True {
                        }
                      }
                    }
                    frame #1 {
                      n247 = case shown="False" w479 {
                        selector: w479 -> [w488 w519]
                        tunnel: [w488 w519] -> w473
                        tunnel: w474 -> [w490 _]
                        tunnel: w478 -> [w483 w518]
                        tunnel: w477 -> [w484 w517]
                        tunnel: [w482 w518] -> w476
                        tunnel: [w481 w517] -> w475
                        frame False {
                          n248 = local read "Gstep"() -> (w486:dbl)
                          n249 = Unbundle By Name(w490) -> ("Data"=w487:u32[], "Data2"=w485:u32[], "HardN"=w492:i32)
                          n250 = Decrement(x=w492) -> (x-1=w491:i32)
                          n251 = local read "Real"() -> (w480:bool)
                          n252 = Equal To 0?(x=w491) -> (x = 0?=w489:bool)
                          n253 = case shown="True" w489 {
                            tunnel: w487 -> [w501 w511]
                            tunnel: w486 -> [w494 w508]
                            tunnel: w485 -> [w500 _]
                            tunnel: w484 -> [w498 w509]
                            tunnel: w483 -> [w497 w510]
                            tunnel: [w496 w509] -> w481
                            tunnel: [w495 w506] -> w482
                            tunnel: w480 -> [w493 w507]
                            frame False {
                              n254 = Build Array (concatenate)(w497, w501) -> (w495:u32[])
                              n255 = Build Array (concatenate)(w498, w500) -> (w496:u32[])
                              n256 = Build Array(w495, w496) -> (w499:u32[][])
                              n257 = case shown="True" w493 {
                                tunnel: w499 -> [_ w504]
                                tunnel: w494 -> [_ w502]
                                frame False {
                                }
                                frame True {
                                n258 = Bundle("y"=0.0, "Gstep"=w502, w504) -> (w503:cluster{"y":dbl, "Gstep":dbl, u32[][]})  [unwired: 1 out]
                                n259 = local write "Graph"(w503) -> ()
                                }
                              }
                            }
                            frame True {
                              n260 = Build Array (concatenate)(w510, w511) -> (w506:u32[])
                              n261 = case shown="True" w507 {
                                tunnel: w508 -> [_ w513]
                                tunnel: w506 -> [_ w512]
                                frame False {
                                }
                                frame True {
                                n262 = Build Array(w512) -> (w515:u32[][])
                                n263 = Bundle("y"=0.0, "Gstep"=w513, w515) -> (w514:cluster{"y":dbl, "Gstep":dbl, u32[][]})  [unwired: 1 out]
                                n264 = local write "Graph"(w514) -> ()
                                }
                              }
                            }
                          }
                        }
                        frame True {
                        }
                      }
                    }
                    frame #2 {
                      n265 = local read "SStop"() -> (w520:bool)
                      n266 = Or(x=w520, y=w521) -> (x .or. y?=w522:bool)
                    }
                  }
                }
              }
              frame #1 {
                n267 = Unbundle By Name(w529) -> ("HardN"=w528:i32)
                n268 = Decrement(x=w528) -> (x-1=w527:i32)
                n269 = Equal To 0?(x=w527) -> (x = 0?=w526:bool)
                n270 = case shown="False" w526 {
                  tunnel: w525 -> [w531 w534]
                  tunnel: w524 -> [w530 _]
                  tunnel: [w532 w533] -> w523
                  frame False {
                    n271 = Build Array(w531, w530) -> (w532:u32[][])
                  }
                  frame True {
                    n272 = Build Array(w534) -> (w533:u32[][])
                  }
                }
              }
            }
            n273 = case shown="True" w445 {
              tunnel: [w535 w538] -> w443
              tunnel: w444 -> [w535 w537]
              frame False {
              }
              frame True {
                n274 = Build Array (concatenate)(w537, "Reset", "WPort") -> (w538:string[])
              }
            }
          }
          frame False {
            n275 = for {
              N: w546 -> [_]
              tunnel: w550 -> [w562]
              shift-right: [w560] -> w548
              shift-left: w549 -> [w561]
              shift-right: [w558] -> w541
              shift-left: u32[][] [] -> [w559]
              shift-right: [w556] -> w544
              shift-left: FALSE ("Error") -> [w557]
              n276 = stacked-sequence {
                seq-local: [w565 _ _] -> [_ w598 _]
                seq-local: [w566 _ _] -> [_ w597 _]
                seq-local: [w564 _ _] -> [_ w594 _]
                seq-local: [_ w594 _] -> [_ _ w623]
                tunnel: w562 -> [w571 _ _]
                tunnel: w561 -> [w568 w599 _]
                tunnel: [w567 _ _] -> w560
                tunnel: w559 -> [_ w595 _]
                tunnel: [_ w596 _] -> w558
                tunnel: w557 -> [w563 _ _]
                tunnel: [_ _ w622] -> w556
                frame #0 {
                  w572 = u32[] []
                  n277 = for {
                    N: w571 -> [_]
                    shift-right: [w579] -> w567
                    shift-left: w568 -> [w580]
                    shift-right: [w578] -> w564
                    shift-left: w563 -> [w577]
                    shift-right: [w574] -> w569
                    shift-left: w572 -> [w573]
                    shift-right: [w576] -> w570
                    shift-left: w572 -> [w575]
                    n278 = case shown="False" w577 {
                      tunnel: w580 -> [w589 w592]
                      tunnel: [w588 w592] -> w579
                      tunnel: [w587 w593] -> w578
                      tunnel: w577 -> [_ w593]
                      tunnel: [w585 w591] -> w576
                      tunnel: w575 -> [w584 w591]
                      tunnel: [w582 w590] -> w574
                      tunnel: w573 -> [w581 w590]
                      frame False {
                        n279 = call "C8855-01_ReadData.vi"("MainD"=w589) -> ("MainDR"=w588:T1, "Error"=w587:bool)  [unwired: 9 out]
                        n280 = Unbundle By Name(w588) -> ("Data"=w586:u32[], "Data2"=w583:u32[])
                        n281 = Build Array (concatenate)(w581, w583) -> (w582:u32[])
                        n282 = Build Array (concatenate)(w584, w586) -> (w585:u32[])
                      }
                      frame True {
                      }
                    }
                  }
                  n283 = Add Array Elements(numeric array=w570) -> (sum=w565:u32)
                  n284 = Add Array Elements(numeric array=w569) -> (sum=w566:u32)
                }
                frame #1 {
                  n285 = case shown="False" w594 {
                    tunnel: w599 -> [w609 _]
                    tunnel: w598 -> [w606 _]
                    tunnel: w597 -> [w605 _]
                    tunnel: [w601 w620] -> w596
                    tunnel: w595 -> [w604 w620]
                    frame False {
                      n286 = Unbundle By Name(w609) -> ("HardN"=w608:i32)
                      n287 = Decrement(x=w608) -> (x-1=w607:i32)
                      n288 = local read "Real"() -> (w600:bool)
                      n289 = Equal To 0?(x=w607) -> (x = 0?=w603:bool)
                      n290 = case shown="False" w603 {
                        tunnel: w606 -> [w616 w619]
                        tunnel: w605 -> [w615 _]
                        tunnel: [w617 w618] -> w602
                        frame False {
                          n291 = Build Array(w616, w615) -> (w617:u32[])
                        }
                        frame True {
                          n292 = Build Array(w619) -> (w618:u32[])
                        }
                      }
                      n293 = Build Array (concatenate)(w604, w602) -> (w601:u32[][])
                      n294 = case shown="True" w600 {
                        tunnel: w601 -> [_ w611]
                        frame False {
                        }
                        frame True {
                          n295 = Transpose 2D Array(2D array=w611) -> (transposed array=w610:u32[][])
                          n296 = local read "Gstep"() -> (w613:dbl)
                          n297 = Bundle("y"=0.0, "Gstep"=w613, w610) -> (w612:cluster{"y":dbl, "Gstep":dbl, u32[][]})  [unwired: 1 out]
                          n298 = local write "Graph"(w612) -> ()
                        }
                      }
                    }
                    frame True {
                    }
                  }
                }
                frame #2 {
                  n299 = local read "SStop"() -> (w621:bool)
                  n300 = Or(x=w621, y=w623) -> (x .or. y?=w622:bool)
                }
              }
            }
            n301 = case shown="True" w544 {
              tunnel: [w553 w555] -> w542
              tunnel: w543 -> [w552 w555]
              frame True {
                n302 = Build Array (concatenate)(w552, "Reset", "WPort") -> (w553:string[])
              }
              frame False {
              }
            }
            n303 = Transpose 2D Array(2D array=w541) -> (transposed array=w540:u32[][])
          }
        }
      }
      frame "Stop" {
        n304 = Unbundle By Name(w630) -> ("Handle"=w626:i64[], "HardN"=w629:i32)
        n305 = Decrement(x=w629) -> (x-1=w628:i32)
        n306 = Not Equal To 0?(x=w628) -> (x != 0?=w627:bool)
        n307 = case shown="False" w627 {
          tunnel: w626 -> [w645 w651]
          tunnel: [w642 w648] -> w625
          frame True {
            n308 = Index Array(array=w645, index=1 ("指標")) -> (element=w647:i64)
            n309 = Index Array(array=w645, index=0 ("指標")) -> (element=w646:i64)
            n310 = dll-call lib="PTH2³unc \\\\den0\\é›»å¿œã‚·ã‚¹ãƒ†ãƒ éƒ¨é›»å¿œã‚·ã‚¹ãƒ†ãƒ éƒ¨å†…è³‡æ–™13éƒ¨é–€33412â–  C8855-01â–¡ä»˜å±žï¼£ï¼¤C8855-01 Ver3.4[æœ€æ–°]SampleSourcex64C8855-01api.dll" fn="C8855CountStop"("Hnadle"=w647) -> ("返り値タイプ"=w640:i32)  [unwired: 4 in, 2 out]
            n311 = dll-call lib="PTH2³unc \\\\den0\\é›»å¿œã‚·ã‚¹ãƒ†ãƒ éƒ¨é›»å¿œã‚·ã‚¹ãƒ†ãƒ éƒ¨å†…è³‡æ–™13éƒ¨é–€33412â–  C8855-01â–¡ä»˜å±žï¼£ï¼¤C8855-01 Ver3.4[æœ€æ–°]SampleSourcex64C8855-01api.dll" fn="C8855CountStop"("Hnadle"=w646) -> ("返り値タイプ"=w641:i32)  [unwired: 4 in, 2 out]
            n312 = Less Or Equal To 0?(x=w641) -> (x <= 0?=w638:bool)
            n313 = Less Or Equal To 0?(x=w640) -> (x <= 0?=w639:bool)
            n314 = Or(x=w638, y=w639) -> (x .or. y?=w642:bool)
          }
          frame False {
            n315 = Index Array(array=w651, index=0 ("指標")) -> (element=w650:i64)
            n316 = dll-call lib="PTH2³unc \\\\den0\\é›»å¿œã‚·ã‚¹ãƒ†ãƒ éƒ¨é›»å¿œã‚·ã‚¹ãƒ†ãƒ éƒ¨å†…è³‡æ–™13éƒ¨é–€33412â–  C8855-01â–¡ä»˜å±žï¼£ï¼¤C8855-01 Ver3.4[æœ€æ–°]SampleSourcex64C8855-01api.dll" fn="C8855CountStop"("Hnadle"=w650) -> ("返り値タイプ"=w649:i32)  [unwired: 4 in, 2 out]
            n317 = Less Or Equal To 0?(x=w649) -> (x <= 0?=w648:bool)
          }
        }
        n318 = case shown="True" w625 {
          frame False {
          }
          frame True {
            n319 = One Button Dialog(message="Error : Stop()\nCheck C8855-01" ("爷景嫁")) -> (true=w636:bool)  [unwired: 1 out]
            n320 = case shown="True" w636 {
              frame False {
              }
              frame True {
                n321 = Quit LabVIEW() -> ()  [unwired: 1 out]
              }
            }
          }
        }
      }
      frame "FinalDisp" {
        n322 = Array Size(array=w653) -> (size(s)=w661:i32[])
        n323 = local read "MP"() -> (w657:u32)
        n324 = To Long Integer(number=w657) -> (32bit integer=w654:i32)
        n325 = Index Array(array=w661, index=1 ("指標")) -> (element=w660:i32)
        n326 = To Unsigned Long Integer(number=w660) -> (unsigned 32bit integer=w659:u32)
        n327 = Greater?(x=w659, y=w657) -> (0:w658:bool)
        n328 = case shown="True" w658 {
          tunnel: w653 -> [w671 w674]
          tunnel: w654 -> [_ w673]
          tunnel: [w671 w672] -> w656
          frame False {
          }
          frame True {
            n329 = Array Subset(array=w674, length (col)=w673) -> (w672:u32[][])  [unwired: 3 in]
          }
        }
        n330 = local read "Gstep"() -> (w663:dbl)
        n331 = Bundle("y"=0.0, "Gstep"=w663, w656) -> (w655:cluster{"y":dbl, "Gstep":dbl, u32[][]})  [unwired: 1 out]
        n332 = local write "Graph"(w655) -> ()
      }
      frame "//////////////////////" {
      }
      frame "MoniSetup" {
        w682 = "0" ("Moni1")
        n333 = Unbundle By Name(w687) -> ("HardN"=w691:i32, "Handle"=w692:i64[])
        n334 = for {
          tunnel: w692 -> [w707] mode=indexing
          n335 = dll-call lib="PTH2³unc \\\\den0\\é›»å¿œã‚·ã‚¹ãƒ†ãƒ éƒ¨é›»å¿œã‚·ã‚¹ãƒ†ãƒ éƒ¨å†…è³‡æ–™13éƒ¨é–€33412â–  C8855-01â–¡ä»˜å±žï¼£ï¼¤C8855-01 Ver3.4[æœ€æ–°]SampleSourcex64C8855-01api.dll" fn="C8855Setup"("Handle"=w707, "Gatetime"=u8 12, "Transmode"=u8 2, "Number of gate"=u16 2) -> ("返り値タイプ"=w704:i32)  [unwired: 7 in, 2 out]
          n336 = Less Or Equal To 0?(x=w704) -> (x <= 0?=w703:bool)
          n337 = case shown="True" w703 {
            frame False {
            }
            frame True {
              n338 = One Button Dialog(message="Error : Setup()\nCheck C8855-01" ("爷景嫁")) -> (true=w709:bool)  [unwired: 1 out]
              n339 = case shown="True" w709 {
                frame False {
                }
                frame True {
                  n340 = Quit LabVIEW() -> ()  [unwired: 1 out]
                }
              }
            }
          }
        }
        n341 = Decrement(x=w691) -> (x-1=w690:i32)
        n342 = case shown="0, Default" w690 {
          tunnel: [TRUE ("表示") TRUE ("表示")] -> w689
          tunnel: [FALSE ("表示") TRUE ("表示")] -> w688
          frame 0, Default {
          }
          frame 1 {
          }
        }
        n343 = property on="Moni1" class="Str"("Visible"=w689) -> ()  [unwired: 2 in, 2 out]
        n344 = property on="Moni2" class="Str"("Visible"=w688) -> ()  [unwired: 2 in, 2 out]
        n345 = local write "Moni1"(w682) -> ()
        n346 = local write "Moni2"(w682) -> ()
        n347 = Initialize Array(u32 0 ("element"), 10 ("次元サイズ")) -> (w683:u32[])
        n348 = Bundle By Name(cluster=w687, "Data"=w683, "Data2"=w683) -> (w686:T1)
      }
      frame "MoniRead" {
        n349 = while {
          tunnel: w711 -> [w718]
          stop <- w719 stop-if-true
          n350 = stacked-sequence {
            seq-local: [w722 _ _] -> [_ w756 w767]
            seq-local: [w723 _ _] -> [_ w757 _]
            seq-local: [w720 _ _] -> [_ w755 w764]
            tunnel: w718 -> [w724 _ _]
            tunnel: [_ _ w767] -> _
            tunnel: [_ _ w765] -> w719
            frame #0 {
              w725 = u32[] []
              n351 = for {
                N: 5 -> [_]
                shift-right: [w733] -> w723
                shift-left: w725 -> [w732]
                shift-right: [w731] -> w722
                shift-left: w725 -> [w730]
                tunnel: w724 -> [w729]
                shift-right: [w727] -> w720
                shift-left: FALSE -> [w728]
                n352 = case shown="False" w728 {
                  selector: w728 -> [_ w754]
                  tunnel: [w739 w753] -> w733
                  tunnel: w732 -> [w738 w753]
                  tunnel: [w737 w752] -> w731
                  tunnel: w730 -> [w736 w752]
                  tunnel: w729 -> [w735 _]
                  tunnel: [w734 w754] -> w727
                  frame False {
                    n353 = stacked-sequence {
                      seq-local: [w740 _] -> [_ w750]
                      tunnel: [w746 _] -> w739
                      tunnel: w738 -> [w745 _]
                      tunnel: [w744 _] -> w737
                      tunnel: w736 -> [w742 _]
                      tunnel: w735 -> [w741 _]
                      tunnel: [_ w749] -> w734
                      frame #0 {
                        n354 = call "C8855-01_ReadData.vi"("MainD"=w741) -> ("MainDR"=w748:T1, "Error"=w740:bool)  [unwired: 9 out]
                        n355 = Unbundle By Name(w748) -> ("Data"=w747:u32[], "Data2"=w743:u32[])
                        n356 = Build Array (concatenate)(w742, w743) -> (w744:u32[])
                        n357 = Build Array (concatenate)(w745, w747) -> (w746:u32[])
                      }
                      frame #1 {
                        n358 = local read "SStop"() -> (w751:bool)
                        n359 = Or(x=w751, y=w750) -> (x .or. y?=w749:bool)
                      }
                    }
                  }
                  frame True {
                  }
                }
              }
            }
            frame #1 {
              n360 = case shown="False" w755 {
                tunnel: w757 -> [w762 _]
                tunnel: w756 -> [w763 _]
                frame False {
                  n361 = Add Array Elements(numeric array=w762) -> (sum=w760:u32)
                  n362 = Add Array Elements(numeric array=w763) -> (sum=w758:u32)
                  n363 = call "C8855-01_NumForming.vi"("In"=w758) -> ("Out"=w759:string)  [unwired: 9 in]
                  n364 = call "C8855-01_NumForming.vi"("In"=w760) -> ("Out"=w761:string)  [unwired: 9 in]
                  n365 = local write "Moni1"(w761) -> ()
                  n366 = local write "Moni2"(w759) -> ()
                }
                frame True {
                }
              }
            }
            frame #2 {
              n367 = local read "SStop"() -> (w766:bool)
              n368 = Or(x=w766, y=w764) -> (x .or. y?=w765:bool)
              n369 = call <vilib>:"Beep.vi"() -> ()  [unwired: 3 in, 9 out]
            }
          }
        }
      }
      frame "*******************" {
      }
      frame "SWOff" {
        w775 = u8 2 ("無効")
        n370 = local read "Monitor"() -> (w776:bool)
        n371 = local read "Start"() -> (w777:bool)
        n372 = Or(x=w777, y=w776) -> (x .or. y?=w778:bool)
        n373 = case shown="True" w778 {
          frame False {
          }
          frame True {
            n374 = local write "SStop"(FALSE ("SStop")) -> ()
            n375 = property on="SStop" class="Bool (strict)"("Visible"=TRUE ("表示")) -> ()  [unwired: 2 in, 2 out]
          }
        }
        n376 = property on="TrgMode" class="Ring (strict)"("DisabledEnum"=w775) -> ()  [unwired: 2 in, 2 out]
        n377 = property on="LIN_Log" class="Bool (strict)"("Disabled"=w775) -> ()  [unwired: 2 in, 2 out]
        n378 = property on="Monitor" class="Bool (strict)"("Disabled"=w775) -> ()  [unwired: 2 in, 2 out]
        n379 = property on="Save" class="Bool (strict)"("Disabled"=w775) -> ()  [unwired: 2 in, 2 out]
        n380 = property on="Exit" class="Bool (strict)"("Disabled"=w775) -> ()  [unwired: 2 in, 2 out]
        n381 = property on="Start" class="Bool (strict)"("Disabled"=w775) -> ()  [unwired: 2 in, 2 out]
        n382 = property on="Tab" class="TabCtl (strict)"("Disabled"=w775) -> ()  [unwired: 2 in, 2 out]
        n383 = property on="GT" class="Ring (strict)"("Disabled"=w775) -> ()  [unwired: 2 in, 2 out]
        n384 = property on="MP" class="DigNum (strict)"("Disabled"=w775) -> ()  [unwired: 2 in, 2 out]
        n385 = property on="Load" class="Bool (strict)"("Disabled"=w775) -> ()  [unwired: 2 in, 2 out]
        n386 = property on="TrgEdge" class="Ring (strict)"("DisabledEnum"=w775) -> ()  [unwired: 2 in, 2 out]
      }
      frame "SWOn" {
        w790 = u8 0 ("無効")
        w793 = FALSE ("Start")
        w792 = FALSE ("表示")
        n387 = local read "Continue"() -> (w791:bool)
        n388 = case shown="True" w791 {
          tunnel: [w801 u8 2 ("無効")] -> w789
          tunnel: [w801 u8 1 ("無効")] -> w788
          frame False {
            w801 = u8 0 ("無効")
          }
          frame True {
          }
        }
        n389 = property on="LIN_Log" class="Bool (strict)"("Disabled"=w790) -> ()  [unwired: 2 in, 2 out]
        n390 = property on="Exit" class="Bool (strict)"("Disabled"=w790) -> ()  [unwired: 2 in, 2 out]
        n391 = property on="Load" class="Bool (strict)"("Disabled"=w790) -> ()  [unwired: 2 in, 2 out]
        n392 = property on="SStop" class="Bool (strict)"("Visible"=w792) -> ()  [unwired: 2 in, 2 out]
        n393 = property on="Monitor" class="Bool (strict)"("Disabled"=w789) -> ()  [unwired: 2 in, 2 out]
        n394 = property on="MP" class="DigNum (strict)"("Disabled"=w788) -> ()  [unwired: 2 in, 2 out]
        n395 = property on="TrgMode" class="Ring (strict)"("DisabledEnum"=w788) -> ()  [unwired: 2 in, 2 out]
        n396 = property on="Moni1" class="Str"("Visible"=w792) -> ()  [unwired: 2 in, 2 out]
        n397 = property on="Start" class="Bool (strict)"("Disabled"=w789) -> ()  [unwired: 2 in, 2 out]
        n398 = property on="GT" class="Ring (strict)"("Disabled"=w788) -> ()  [unwired: 2 in, 2 out]
        n399 = property on="TrgEdge" class="Ring (strict)"("DisabledEnum"=w788) -> ()  [unwired: 2 in, 2 out]
        n400 = property on="Moni2" class="Str"("Visible"=w792) -> ()  [unwired: 2 in, 2 out]
        n401 = local write "Start"(w793) -> ()
        n402 = local write "Monitor"(w793) -> ()
        n403 = property on="Tab" class="TabCtl (strict)"("Disabled"=w789) -> ()  [unwired: 2 in, 2 out]
        n404 = local write "Save"(w793) -> ()
        n405 = local write "Load"(w793) -> ()
        n406 = property on="Save" class="Bool (strict)"("Disabled"=w789) -> ()  [unwired: 2 in, 2 out]
      }
      frame "PMTPower" {
        n407 = local read "Power"() -> (w809:bool)
        n408 = local read "Power2"() -> (w808:bool)
        n409 = Boolean To (0,1)(Boolean=w809) -> (0, 1=w807:i16)
        n410 = Boolean To (0,1)(Boolean=w808) -> (0, 1=w806:i16)
        n411 = Build Array(w807, w806) -> (w805:i16[])
        n412 = Unbundle By Name(w811) -> ("Handle"=w810:i64[])
        n413 = To Unsigned Byte Integer(number=w805) -> (unsigned 8bit integer=w804:u8[])
        n414 = for {
          tunnel: w810 -> [w821] mode=indexing
          tunnel: w804 -> [w820] mode=indexing
          n415 = dll-call lib="PTH2³unc \\\\den0\\é›»å¿œã‚·ã‚¹ãƒ†ãƒ éƒ¨é›»å¿œã‚·ã‚¹ãƒ†ãƒ éƒ¨å†…è³‡æ–™13éƒ¨é–€33412â–  C8855-01â–¡ä»˜å±žï¼£ï¼¤C8855-01 Ver3.4[æœ€æ–°]SampleSourcex64C8855-01api.dll" fn="C8855SetPmtPower"("Hnadle"=w821, "Power State"=w820) -> ("返り値タイプ"=w819:i32)  [unwired: 5 in, 2 out]
          n416 = Less Or Equal To 0?(x=w819) -> (x <= 0?=w818:bool)
          n417 = case shown="True" w818 {
            frame False {
            }
            frame True {
              n418 = One Button Dialog(message="Error : PMTPower()\nCheck C8855-01" ("爷景嫁")) -> (true=w822:bool)  [unwired: 1 out]
              n419 = case shown="True" w822 {
                frame False {
                }
                frame True {
                  n420 = Quit LabVIEW() -> ()  [unwired: 1 out]
                }
              }
            }
          }
        }
      }
      frame "PowerOFF" {
        n421 = Unbundle By Name(w825) -> ("Handle"=w824:i64[])
        n422 = for {
          tunnel: w824 -> [w835] mode=indexing
          n423 = dll-call lib="PTH2³unc \\\\den0\\é›»å¿œã‚·ã‚¹ãƒ†ãƒ éƒ¨é›»å¿œã‚·ã‚¹ãƒ†ãƒ éƒ¨å†…è³‡æ–™13éƒ¨é–€33412â–  C8855-01â–¡ä»˜å±žï¼£ï¼¤C8855-01 Ver3.4[æœ€æ–°]SampleSourcex64C8855-01api.dll" fn="C8855SetPmtPower"("Hnadle"=w835, "Power State"=u8 0) -> ("返り値タイプ"=w833:i32)  [unwired: 5 in, 2 out]
          n424 = Less Or Equal To 0?(x=w833) -> (x <= 0?=w832:bool)
          n425 = case shown="True" w832 {
            frame False {
            }
            frame True {
              n426 = One Button Dialog(message="Error : PMTPower()\nCheck C8855-01" ("爷景嫁")) -> (true=w836:bool)  [unwired: 1 out]
              n427 = case shown="True" w836 {
                frame False {
                }
                frame True {
                  n428 = Quit LabVIEW() -> ()  [unwired: 1 out]
                }
              }
            }
          }
        }
      }
      frame "WPort" {
        n429 = stacked-sequence {
          seq-local: [w845 _] -> [_ w861]
          tunnel: w838 -> [_ w862]
          frame #0 {
            n430 = local read "OP10"() -> (w860:bool)
            n431 = local read "OP11"() -> (w859:bool)
            n432 = local read "OP20"() -> (w849:bool)
            n433 = local read "OP21"() -> (w850:bool)
            n434 = Boolean To (0,1)(Boolean=w860) -> (0, 1=w855:i16)
            n435 = Boolean To (0,1)(Boolean=w859) -> (0, 1=w858:i16)
            n436 = Boolean To (0,1)(Boolean=w849) -> (0, 1=w851:i16)
            n437 = Boolean To (0,1)(Boolean=w850) -> (0, 1=w854:i16)
            n438 = Multiply(x=i16 2, y=w858) -> (x*y=w856:i16)
            n439 = Multiply(x=i16 2, y=w854) -> (x*y=w852:i16)
            n440 = Add(x=w855, y=w856) -> (x+y=w848:i16)
            n441 = Add(x=w851, y=w852) -> (x+y=w847:i16)
            n442 = Build Array(w848, w847) -> (w846:i16[])
            n443 = To Unsigned Byte Integer(number=w846) -> (unsigned 8bit integer=w845:u8[])
          }
          frame #1 {
            n444 = Unbundle By Name(w862) -> ("Handle"=w863:i64[])
            n445 = for {
              tunnel: w863 -> [w867] mode=indexing
              tunnel: w861 -> [w866] mode=indexing
              n446 = dll-call lib="PTH2³unc \\\\den0\\é›»å¿œã‚·ã‚¹ãƒ†ãƒ éƒ¨é›»å¿œã‚·ã‚¹ãƒ†ãƒ éƒ¨å†…è³‡æ–™13éƒ¨é–€33412â–  C8855-01â–¡ä»˜å±žï¼£ï¼¤C8855-01 Ver3.4[æœ€æ–°]SampleSourcex64C8855-01api.dll" fn="C8855WritePort"("Hnadle"=w867, "Data"=w866) -> ("返り値タイプ"=w865:i32)  [unwired: 5 in, 2 out]
              n447 = Less Or Equal To 0?(x=w865) -> (x <= 0?=w864:bool)
              n448 = case shown="True" w864 {
                frame False {
                }
                frame True {
                  n449 = One Button Dialog(message="Error : WritePort()\nCheck C8855-01" ("爷景嫁")) -> (true=w868:bool)  [unwired: 1 out]
                  n450 = case shown="True" w868 {
                    frame False {
                    }
                    frame True {
                      n451 = Quit LabVIEW() -> ()  [unwired: 1 out]
                    }
                  }
                }
              }
            }
          }
        }
      }
      frame "SaveData" {
        n452 = local read "Graph"() -> (w876:cluster{dbl, dbl, u32[][]})
        n453 = Unbundle(w876) -> (w872:dbl, w871:u32[][])  [unwired: 1 out]
        n454 = Array Size(array=w871) -> (size(s)=w875:i32[])
        n455 = Index Array(array=w875, index=1 ("指標")) -> (element=w870:i32)
        n456 = Equal To 0?(x=w870) -> (x = 0?=w873:bool)
        n457 = case shown="False" w873 {
          tunnel: w870 -> [w886 _]
          tunnel: w872 -> [w885 _]
          tunnel: w871 -> [w884 _]
          frame False {
            n458 = stacked-sequence {
              seq-local: [w888 _] -> [_ w898]
              seq-local: [w887 _] -> [_ w897]
              tunnel: w886 -> [_ w907]
              tunnel: w885 -> [_ w906]
              tunnel: w884 -> [_ w905]
              frame #0 {
                n459 = Two Button Dialog(message="Select format ....." ("メッセージ"), 1:"CSV" ("Fボタン名(\"キャンセル\")"), 2:"TAB" ("Tボタン名(\"OK\")")) -> (T button?=w889:bool)
                n460 = case shown="True" w889 {
                  tunnel: ["," "\t"] -> w888
                  tunnel: ["*.csv" ("pattern") "*.xls" ("pattern")] -> w887
                  frame False {
                  }
                  frame True {
                  }
                }
              }
              frame #1 {
                n461 = To Double Precision Float(number=w905) -> (double precision float=w902:dbl[][])
                n462 = for {
                  N: w907 -> [_]
                  tunnel: w906 -> [w910]
                  tunnel: [w908] -> w900 mode=indexing
                  i -> [w911]
                  n463 = To Double Precision Float(number=w911) -> (double precision float=w909:dbl)
                  n464 = Multiply(x=w910, y=w909) -> (x*y=w908:dbl)
                }
                n465 = Build Array (concatenate)(w900, w902) -> (w904:dbl[][])
                n466 = To Single Precision Float(number=w904) -> (single precision float=w901:sgl[][])
                n467 = Transpose 2D Array(2D array=w901) -> (transposed array=w899:sgl[][])
                n468 = call "C8855-01_WriteToSpreadsheetFile.vi"("delimiter (Tab)"=w898, "format (%.3f)"="%.5f", "pattern"=w897, "2D data"=w899) -> ()  [unwired: 4 in, 4 out]
              }
            }
          }
          frame True {
            n469 = call <vilib>:"Beep.vi"() -> ()  [unwired: 3 in, 9 out]
            n470 = One Button Dialog(message="Nothing Data" ("メッセージ")) -> ()  [unwired: 2 out]
          }
        }
      }
      frame "LoadData" {
        n471 = Two Button Dialog(message="Select format ....." ("メッセージ"), 1:"CSV" ("Fボタン名(\"キャンセル\")"), 2:"TAB" ("Tボタン名(\"OK\")")) -> (T button?=w916:bool)
        n472 = case shown="False" w916 {
          tunnel: ["," "\t"] -> w915
          tunnel: ["*.csv" ("[pattern]") "*.xls" ("[pattern]")] -> w914
          frame False {
          }
          frame True {
          }
        }
        n473 = call "C8855-01_ReadFromSpreadsheetFile.vi"("[pattern]"=w914, "delimiter (Tab)"=w915) -> ("new file path (Not A Path if cancelled)"=w925:path, "all rows"=w923:sgl[][])  [unwired: 4 in, 8 out]
        n474 = Equal?(x=w925, y=path "") -> (x = y?=w924:bool)
        n475 = Transpose 2D Array(2D array=w923) -> (transposed array=w922:sgl[][])
        n476 = case shown="False" w924 {
          tunnel: w922 -> [w946 _]
          tunnel: [w944 w956] -> w921
          tunnel: w920 -> [_ w956]
          tunnel: w913 -> [w937 _]
          frame False {
            n477 = Array Size(array=w946) -> (size(s)=w953:i32[])
            n478 = Index Array(array=w946, index (row)=0 ("指標 （行）"), index (col)=1 ("無効な指標 （列）")) -> (element=w948:sgl)
            n479 = Index Array(array=w953, index=0 ("指標")) -> (element=w951:i32)
            n480 = Index Array(array=w953, index=1 ("指標")) -> (element=w954:i32)
            n481 = To Double Precision Float(number=w948) -> (double precision float=w938:dbl)
            n482 = Decrement(x=w951) -> (x-1=w943:i32)
            n483 = To Unsigned Long Integer(number=w954) -> (unsigned 32bit integer=w942:u32)
            n484 = To Long Integer(number=w942) -> (32bit integer=w939:i32)
            n485 = Array Subset(array=w946, index (row)=1 ("指標"), length (row)=w943, length (col)=w939) -> (w947:sgl[][])  [unwired: 1 in]
            n486 = local write "Gstep"(w938) -> ()
            n487 = call "C8855-01_MakingGate.vi"("MainD"=w937, "GStep"=w938) -> ("StepGate"=w936:i32)  [unwired: 9 out]
            n488 = To Unsigned Long Integer(number=w947) -> (unsigned 32bit integer=w944:u32[][])
            n489 = local write "MP"(w942) -> ()
            n490 = local write "GT"(w936) -> ()
            n491 = To Double Precision Float(number=w942) -> (double precision float=w941:dbl)
            n492 = Multiply(x=w938, y=w941) -> (x*y=w940:dbl)
            n493 = local write "MT"(w940) -> ()
          }
          frame True {
          }
        }
      }
      frame "Plus Windows" {
      }
      frame "*******" {
      }
      frame "Quit" {
        n494 = stacked-sequence {
          tunnel: w971 -> [w979 _]
          frame #0 {
            n495 = local read "Continue"() -> (w978:bool)
            n496 = call "C8855-01_Close.vi"("MainD"=w979, "Continue"=w978) -> ()  [unwired: 10 out]
          }
          frame #1 {
            n497 = Stop() -> ()  [unwired: 1 out]
          }
        }
      }
      frame "Developer Error", Default {
        n498 = call <vilib>:"Beep.vi"() -> ()  [unwired: 3 in, 9 out]
        n499 = Index Array(array=w984) -> (element=w985:string)  [unwired: 1 in]
        n500 = Concatenate Strings(w985, "\r\n", "Error !\nBad Case Name.....\nCheck Program......." ("文字列")) -> (w981:string)
        n501 = One Button Dialog(message=w981) -> (true=w980:bool)  [unwired: 1 out]
        n502 = stacked-sequence {
          tunnel: w980 -> [_]
          frame #0 {
            n503 = Stop() -> ()  [unwired: 1 out]
          }
        }
      }
      frame "Exit" {
        n504 = stacked-sequence {
          tunnel: w992 -> [w1000 _]
          frame #0 {
            n505 = local read "Continue"() -> (w999:bool)
            n506 = call "C8855-01_Close.vi"("MainD"=w1000, "Continue"=w999) -> ()  [unwired: 10 out]
          }
          frame #1 {
            n507 = Quit LabVIEW() -> ()  [unwired: 1 out]
          }
        }
      }
    }
    n508 = call "C8855-01_CaseErase.vi"("Input"=w6) -> ("Output"=w5:string[])  [unwired: 10 out]
  }
